vi "oa_TV Set Channel Info (Waveform Output 1Chan).vi"(4 "output interval [s]":dbl, 6 "t0":dbl, 7 "torisional vibration unit (RPM)":enum16{"RPM", "deg/s", "rad/s"}(ring), 8 "error in (no error)":errorcluster, 9 "pulse position":dbl[](array[numeric]), 10 "seconds/rev":dbl[](array[numeric]) format="%.2f", 11 "revolutions/sec":dbl[](array[numeric]) format="%.2f") -> (0 "error out":errorcluster, 1 "unit label":string, 2 "speed profile":T1 {"speed [RPM]" format="%.2f"; "time [s]" format="%.2f"}, 3 "torsional vibration":waveform(dbl))   [LabVIEW 2017, in "SoundVib_Torsional.lvlib"]
uses:
  <vilib>/addons/Sound and Vibration/Order Analysis/Torsional Vibration/SoundVib_Torsional.lvlib
  <vilib>/addons/Sound and Vibration/Order Analysis/Tach Process/SubVIs/speed profile.ctl
  <vilib>/addons/_NISVFA/_Shared subVIs/Controls/svc_Engineering Units Text Ring.ctl
  <vilib>/addons/_NISVFA/_Shared subVIs/Common/svc_Set SV Channel Info (variant).vi
  <vilib>/addons/_NISVFA/_Shared subVIs/Common/SVL Set dB Reference (variant).vi
  <vilib>/addons/_NISVFA/_Shared subVIs/Common/svc_Engineering Units to Unit Label.vi
  <vilib>/addons/Sound and Vibration/Order Analysis/Tach Process/SoundVib_TachProcess.lvlib
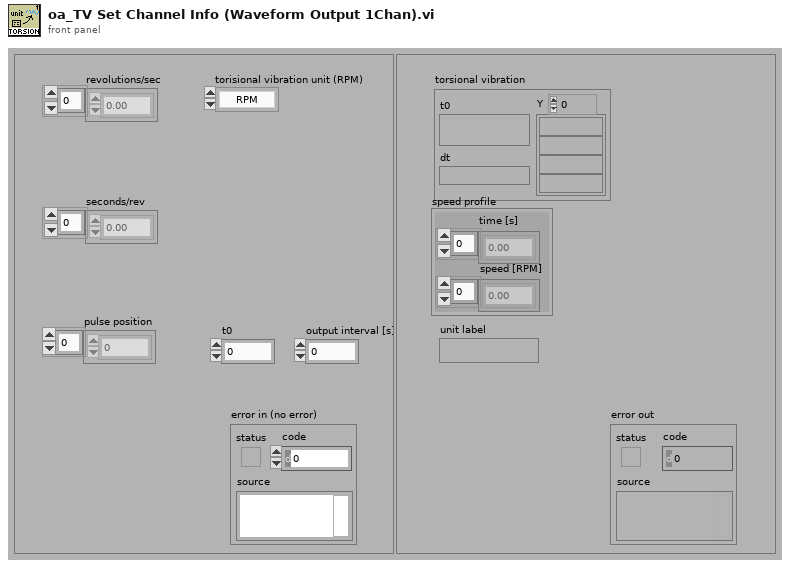
[diagram p1: front panel]
types:
  T1 = typedef "SoundVib_TachProcess.lvlib/speed profile.ctl" = cluster{"time [s]":dbl[], "speed [RPM]":dbl[]}
  T2 = typedef "svc_Engineering Units Text Ring.ctl" = u16
  T3 = typedef "svc_Channel Info.ctl" = cluster{"sensor sensitivity":dbl, "engineering units":T2, "dB reference":dbl, "custom label":string, "weighting filter":T4, "pregain":dbl}
  T4 = typedef "svc_Weighting Filter Text Ring.ctl" = u16
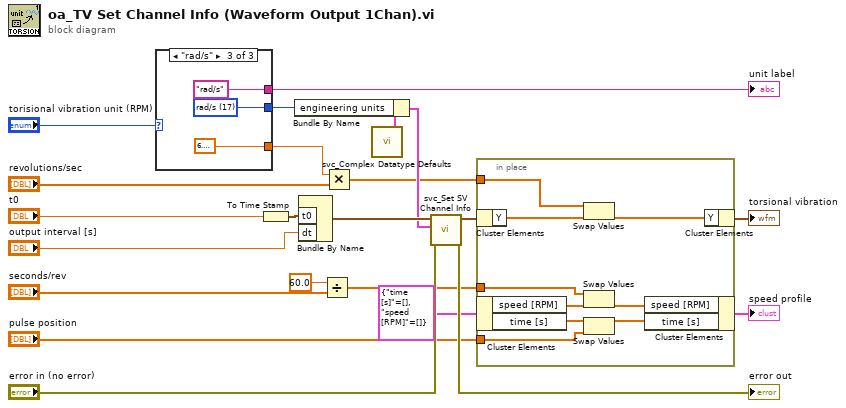
[diagram p0: block diagram]
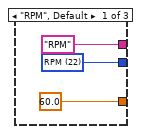
[diagram p2: hidden frame]
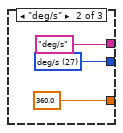
[diagram p3: hidden frame]
diagram:
  n1 = case shown="\"rad/s\"" "torisional vibration unit (RPM)" {
    tunnel: [60.0 ("even-time") 360.0 ("even-time") 6.283185307179586] -> w18
    tunnel: ["RPM" "deg/s" "rad/s"] -> w14
    tunnel: [w23 w26 w29] -> w13
    frame "RPM", Default {
      w23 = T2 22 items=["custom..."=0, "V"=1, "A"=21, "Pa"=2, "N"=20, "g"=3, "m/s^2"=4, "m/s"=5, "m"=6, "mm/s"=12, "mm"=13, "micron/s"=14, "micron"=15, "in/s^2"=7, "in/s"=8, "in"=9, "mil/s"=10, "mil"=11, "rad/s^2"=16, "rad/s"=17, "rad"=18, "deg/s^2"=26, "deg/s"=27, "deg"=28, "RPM"=22, "cycle/s^2"=23, "Hz"=24, "cycle"=25, "strain"=19] ("engineering units")
    }
    frame "deg/s" {
      w26 = T2 27 items=["custom..."=0, "V"=1, "A"=21, "Pa"=2, "N"=20, "g"=3, "m/s^2"=4, "m/s"=5, "m"=6, "mm/s"=12, "mm"=13, "micron/s"=14, "micron"=15, "in/s^2"=7, "in/s"=8, "in"=9, "mil/s"=10, "mil"=11, "rad/s^2"=16, "rad/s"=17, "rad"=18, "deg/s^2"=26, "deg/s"=27, "deg"=28, "RPM"=22, "cycle/s^2"=23, "Hz"=24, "cycle"=25, "strain"=19] ("engineering units")
    }
    frame "rad/s" {
      w29 = T2 17 items=["custom..."=0, "V"=1, "A"=21, "Pa"=2, "N"=20, "g"=3, "m/s^2"=4, "m/s"=5, "m"=6, "mm/s"=12, "mm"=13, "micron/s"=14, "micron"=15, "in/s^2"=7, "in/s"=8, "in"=9, "mil/s"=10, "mil"=11, "rad/s^2"=16, "rad/s"=17, "rad"=18, "deg/s^2"=26, "deg/s"=27, "deg"=28, "RPM"=22, "cycle/s^2"=23, "Hz"=24, "cycle"=25, "strain"=19] ("engineering units")
    }
  }
  "unit label" <- w14
  n2 = To Time Stamp(1:"t0") -> (0:w22:timestamp)
  n3 = Bundle By Name("t0"=w22, "dt"="output interval [s]") -> (w11:waveform(dbl))  [unwired: 1 in]
  n4 = Divide(x=60.0 ("even-time"), y="seconds/rev") -> (x/y=w5:dbl[])
  n5 = Multiply(x=w18, y="revolutions/sec") -> (x*y=w2:dbl[])
  n6 = call <vilib>:"svc_Complex Datatype Defaults.vi"() -> ("channel info"=w12:T3)  [unwired: 11 in, 8 out]
  n7 = Bundle By Name(cluster=w12, "engineering units"=w13) -> (w10:T3)
  n8 = call <vilib>:"svc_Set SV Channel Info.vi"("error in (no error)"="error in (no error)", "channel info"=w10, "scaled signal in"=w11) -> ("error out"=→"error out":errorcluster, "scaled signal out"=w3:waveform(dbl))  [unwired: 7 in]
  n9 = in-place {
    in-place-border: "pulse position" -> [w32]
    in-place-border: w5 -> [w36]
    in-place-border: w2 -> [w38]
    n10 = in-place-cluster #1(w3) -> ("Y"=w40:dbl[])
    n11 = in-place-cluster #2(T1 {"time [s]"=[], "speed [RPM]"=[]} ("speed profile")) -> ("speed [RPM]"=w37:dbl[], "time [s]"=w34:dbl[])
    n12 = Swap Values(12:w38, 14:w40) -> (3:w39:dbl[])  [unwired: 1 in, 1 out]
    n13 = Swap Values(12:w36, 14:w37) -> (3:w35:dbl[])  [unwired: 1 in, 1 out]
    n14 = Swap Values(12:w34, 14:w32) -> (1:w33:dbl[])  [unwired: 1 in, 1 out]
    n15 = in-place-cluster #2("speed [RPM]"=w35, "time [s]"=w33) -> (→"speed profile":T1)
    n16 = in-place-cluster #1("Y"=w39) -> (→"torsional vibration":waveform(dbl))
  }
